vi "moveabs.vi"(2 "SetPosition":sgl format="%.2f", 3 "EXP300 -3A Axis":i8=1, 4 "ESP300 -3A Add.":i32=3) -> ()   [LabVIEW 2010]
panel:
  out "Current Position":dbl
  out "Time to wait (s)":i16
  # "Stage Moving"
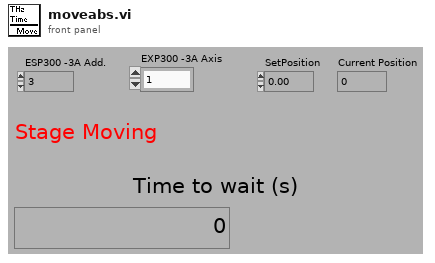
[diagram p1: front panel]
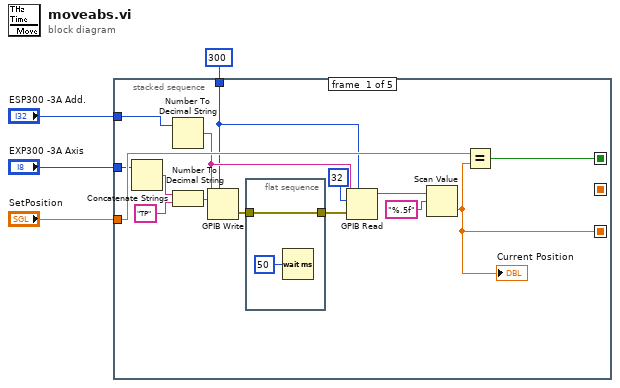
[diagram p0: block diagram]
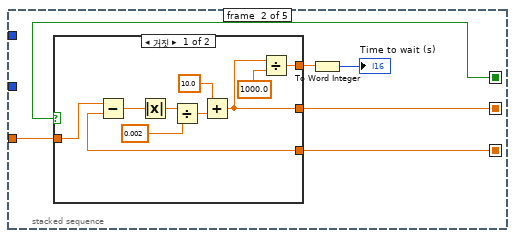
[diagram p2: hidden frame]
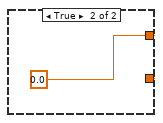
[diagram p3: hidden frame]
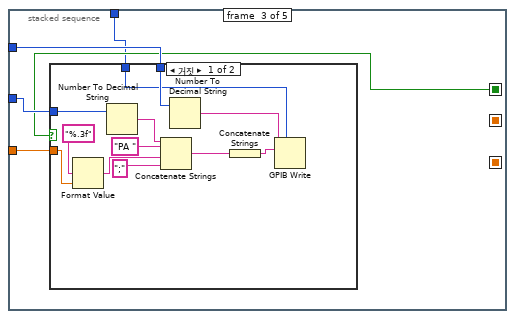
[diagram p4: hidden frame]
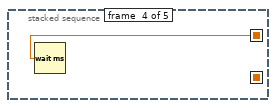
[diagram p6: hidden frame]
diagram:
  n1 = stacked-sequence {
    seq-local: [w18 _ _ _ _] -> [_ w26 _ _ _]
    seq-local: [w16 _ _ _ _] -> [_ w25 w40 _ _]
    seq-local: [_ w24 _ _ _] -> [_ _ _ w56 _]
    tunnel: "ESP300 -3A Add." -> [w15 _ w43 _ _]
    tunnel: "EXP300 -3A Axis" -> [w11 _ w42 _ _]
    tunnel: "SetPosition" -> [w17 w27 w41 _ _]
    tunnel: 300 ("timeout ms (488.2 global)") -> [w9 _ w39 _ _]
    frame #0 {
      n2 = Number To Decimal String(number=w11) -> (decimal integer string=w7:string)  [unwired: 1 in]
      n3 = Number To Decimal String(number=w15) -> (decimal integer string=w13:string)  [unwired: 1 in]
      n4 = Concatenate Strings(w7, "TP" ("string")) -> (w10:string)
      n5 = GPIB Write(0:w13, 1:w10, 4:w9) -> (6:w6:errorcluster)  [unwired: 2 in, 1 out]
      n6 = flat-sequence {
        tunnel: w6 -> [w21]
        tunnel: [w21] -> w5
        frame #0 {
          n7 = Wait (ms)(milliseconds to wait=u32 50) -> ()  [unwired: 1 out]
        }
      }
      n8 = GPIB Read(0:w13, 1:32 ("byte count"), 3:w5, 4:w9) -> (5:w14:string)  [unwired: 1 in, 2 out]
      n9 = Scan Value(string=w14, format string="%.5f") -> (value=w18:dbl)  [unwired: 1 in, 1 out]
      "Current Position" <- w18
      n10 = Equal?(x=w17, y=w18) -> (x = y?=w16:bool)
    }
    frame #1 {
      n11 = case shown="거짓" w25 {
        tunnel: w27 -> [w34 _]
        tunnel: w26 -> [w33 _]
        tunnel: [w29 w38] -> w23
        tunnel: [w28 w38] -> w24
        frame False {
          n12 = Subtract(x=w34, y=w33) -> (x-y=w35:dbl)
          n13 = Absolute Value(x=w35) -> (abs(x)=w36:dbl)
          n14 = Divide(x=w36, y=0.002) -> (x/y=w32:dbl)
          n15 = Add(x=10.0, y=w32) -> (x+y=w28:dbl)
          n16 = Divide(x=w28, y=1000.0) -> (x/y=w29:dbl)
        }
        frame True {
          w38 = 0.0
        }
      }
      n17 = To Word Integer(number=w23) -> (16bit integer=→"Time to wait (s)":i16)
    }
    frame #2 {
      n18 = case shown="거짓" w40 {
        tunnel: w43 -> [w55 _]
        tunnel: w42 -> [w53 _]
        tunnel: w41 -> [w51 _]
        tunnel: w39 -> [w48 _]
        frame False {
          n19 = Format Value(format string="%.3f", value (0)=w51) -> (output string=w50:string)  [unwired: 1 in]
          n20 = Number To Decimal String(number=w53) -> (decimal integer string=w46:string)  [unwired: 1 in]
          n21 = Concatenate Strings(w46, "PA " ("string"), w50, ";" ("string")) -> (w45:string)
          n22 = Number To Decimal String(number=w55) -> (decimal integer string=w54:string)  [unwired: 1 in]
          n23 = Concatenate Strings(w45) -> (w44:string)
          n24 = GPIB Write(0:w54, 1:w44, 4:w48) -> ()  [unwired: 2 in, 2 out]
        }
        frame True {
        }
      }
    }
    frame #3 {
      n25 = Wait (ms)(milliseconds to wait=w56) -> ()  [unwired: 1 out]
    }
    frame #4 {
    }
  }
